vi "Write Numeric.vi"(10 "Numeric":dbl, 11 "Increment Msg in":refnum<class "Increment Msg.lvclass">) -> (3 "Increment Msg out":refnum<class "Increment Msg.lvclass">)   [LabVIEW 2020, in "Messaging Tests.lvlib" / "Increment Msg.lvclass"]
uses:
  Increment Msg.lvclass
  Increment Msg.lvclass/Increment Msg.ctl
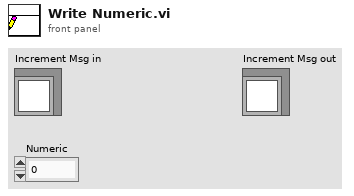
[diagram p1: front panel]
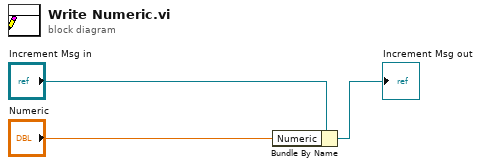
[diagram p0: block diagram]
diagram:
  n1 = Bundle By Name(cluster="Increment Msg in", "Numeric"="Numeric") -> (→"Increment Msg out":refnum<class "Increment Msg.lvclass">)
